vi "FindRouteExample.vi"() -> ()   [LabVIEW 2010]
uses:
  PathTree/RouteTree.lvclass
  Waypoint/point.ctl
  Waypoint/Waypoint.lvclass
panel:
  out "BestTime":u32 caption="Time (ms)"
  out "Best Distance":dbl caption="Distance"
  in  "Best Solve":bool
  out "SmartTime":u32 caption="Time (ms)"
  out "Smart Distance":dbl caption="Distance"
  in  "Smart Solve":bool
  out "FastTime":u32 caption="Time (ms)"
  out "Fast Distance":dbl caption="Distance"
  in  "Fast Solve":bool
  in  "NumPoints":i32
  in  "NewPoints":bool
  in  "Exit":bool
  out "Paths":picture
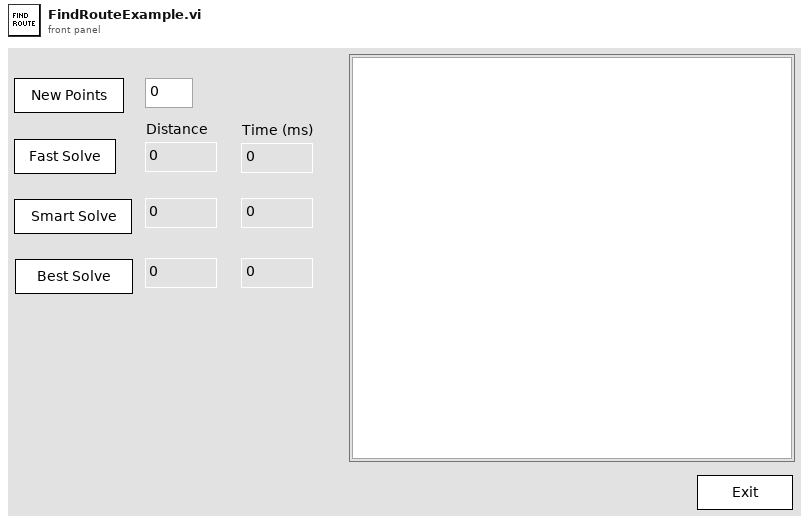
[diagram p1: front panel]
types:
  T1 = typedef "Waypoint.lvclass/point.ctl" = cluster{"X":dbl, "Y":dbl}
  T2 = cluster{"Width":u16, "Style":enum32{"Solid", "Dash", "Dot", "DashDot", "DashDotDot"}}
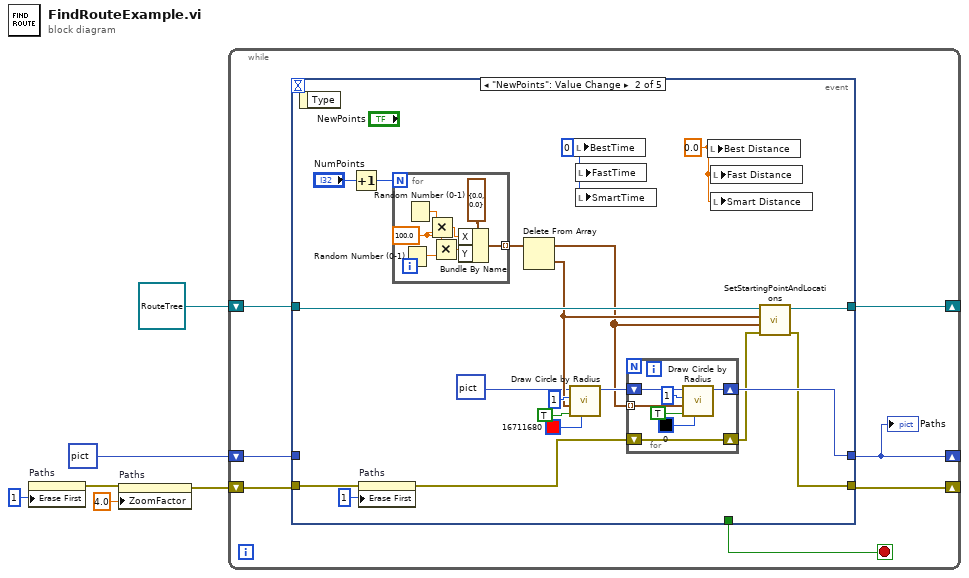
[diagram p0: block diagram]
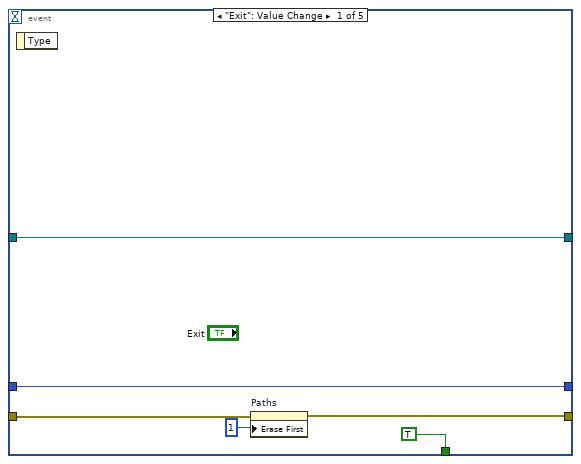
[diagram p2: hidden frame]
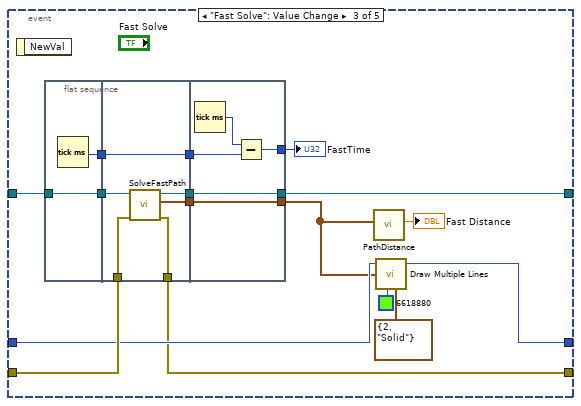
[diagram p3: hidden frame]
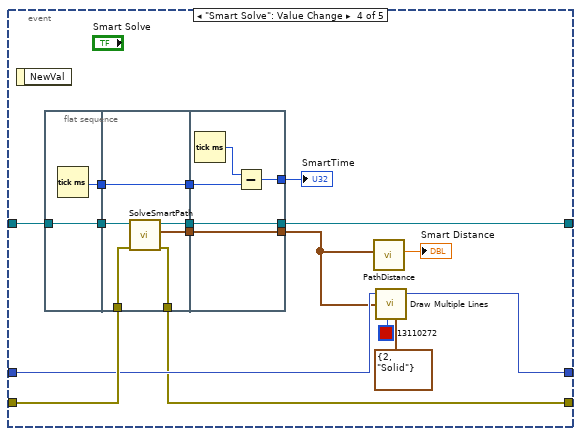
[diagram p4: hidden frame]
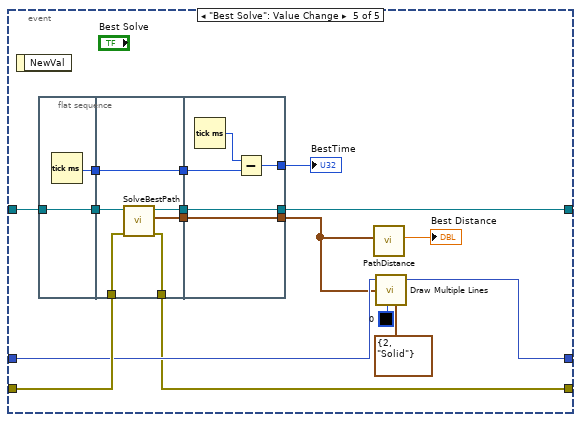
[diagram p5: hidden frame]
diagram:
  n1 = property on="Paths" class="Pict"("Erase First"=u8 1) -> (error out=w1:errorcluster)  [unwired: 2 in, 1 out]
  n2 = property on="Paths" class="Pict"(error in=w1, "ZoomFactor"=sgl 4.0 ("Zoom Factor")) -> (error out=w4:errorcluster)  [unwired: 1 in, 1 out]
  n3 = while {
    shift-right: [w7] -> _
    shift-left: picture data[5B] ("Paths") -> [w10]
    shift-right: [w8] -> _
    shift-left: w4 -> [w9]
    shift-right: [w12] -> _
    shift-left: refnum<class "RouteTree.lvclass"> refnum ("RouteTree.lvclass") -> [w13]
    stop <- w11 stop-if-true
    n4 = event shown="[1] \"NewPoints\": Value Change" {
      selector: _ -> [_ _ _ _ _]
      dyn-events: _ -> [_ _ _ _ _]
      timeout: _ -> [_ _ _ _ _]
      tunnel: w13 -> [w19 w28 w69 w98 w127]
      tunnel: [w19 w27 w68 w97 w126] -> w12
      tunnel: [TRUE _ _ _ _] -> w11
      tunnel: w10 -> [w17 _ w66 w95 w124]
      tunnel: [w17 w29 w63 w92 w121] -> w7
      tunnel: w9 -> [w16 w31 w67 w96 w125]
      tunnel: [w14 w23 w62 w91 w120] -> w8
      event "Exit": Value Change {
        n5 = event-data() -> ()  [unwired: 1 in, 1 out]
        n6 = property on="Paths" class="Pict"(error in=w16, "Erase First"=u8 1) -> (error out=w14:errorcluster)  [unwired: 1 in, 1 out]
      }
      event "NewPoints": Value Change {
        w20 = 0.0 ("Best Distance")
        w21 = u32 0 ("BestTime")
        n7 = event-data() -> ()  [unwired: 1 in, 1 out]
        n8 = Increment(x="NumPoints") -> (x+1=w39:i32)
        n9 = property on="Paths" class="Pict"(error in=w31, "Erase First"=u8 1) -> (error out=w30:errorcluster)  [unwired: 1 in, 1 out]
        n10 = for {
          N: w39 -> [_]
          tunnel: [w47] -> w37 mode=indexing
          w49 = 100.0 ("x")
          n11 = Random Number (0-1)() -> (number: 0 to 1=w51:dbl)
          n12 = Random Number (0-1)() -> (number: 0 to 1=w53:dbl)
          n13 = Multiply(x=w53, y=w49) -> (x*y=w52:dbl)
          n14 = Multiply(x=w49, y=w51) -> (x*y=w50:dbl)
          n15 = Bundle By Name(cluster=T1 {"X"=0.0, "Y"=0.0} ("point"), "X"=w52, "Y"=w50) -> (w47:T1)
        }
        n16 = Delete From Array(array=w37) -> (deleted portion=w26:T1, array with subset deleted=w25:T1[])  [unwired: 2 in]
        n17 = call <vilib>:"Draw Circle by Radius.vi"("color(black)"=u32 16711680, "fill?(F)"=TRUE, "pixel center"=w26, "radius"=i16 1, "picture"=picture data[5B]) -> ("new picture"=w33:picture)  [unwired: 6 in]
        n18 = local write "BestTime"(w21) -> ()
        n19 = local write "FastTime"(w21) -> ()
        n20 = local write "SmartTime"(w21) -> ()
        n21 = for {
          shift-right: [w42] -> w29
          shift-left: w33 -> [w43]
          shift-right: [w41] -> w24
          shift-left: w30 -> [w41]
          tunnel: w25 -> [w40] mode=indexing
          n22 = call <vilib>:"Draw Circle by Radius.vi"("color(black)"=u32 0, "fill?(F)"=TRUE, "pixel center"=w40, "radius"=i16 1, "picture"=w43) -> ("new picture"=w42:picture)  [unwired: 6 in]
        }
        n23 = local write "Best Distance"(w20) -> ()
        n24 = local write "Fast Distance"(w20) -> ()
        n25 = local write "Smart Distance"(w20) -> ()
        n26 = call "SetStartingPointAndLocations.vi"("error in (no error)"=w24, "locations"=w25, "point"=w26, "PathTree in"=w28) -> ("error out"=w23:errorcluster, "PathTree out"=w27:refnum<class "RouteTree.lvclass">)  [unwired: 6 in]
      }
      event "Fast Solve": Value Change {
        n27 = event-data() -> ()  [unwired: 1 in, 1 out]
        n28 = flat-sequence {
          tunnel: w69 -> [w71]
          tunnel: [w71] -> w57
          tunnel: [w70] -> w56
          tunnel: w67 -> [w75]
          tunnel: [w74] -> w62
          tunnel: [w76] -> w59
          tunnel: [w73] -> w58
          tunnel: w57 -> [w77]
          tunnel: w56 -> [w72]
          tunnel: [w72] -> w55
          tunnel: [w81] -> w61
          tunnel: [w82] -> w68
          tunnel: w59 -> [w82]
          tunnel: w58 -> [w81]
          tunnel: w55 -> [w79]
          tunnel: [w78] -> w54
          frame #0 {
            n29 = Tick Count (ms)() -> (millisecond timer value=w70:u32)
          }
          frame #1 {
            n30 = call "SolveFastPath.vi"("error in (no error)"=w75, "RouteTree in"=w77) -> ("error out"=w74:errorcluster, "greedy Path"=w73:T1[], "RouteTree out"=w76:refnum<class "RouteTree.lvclass">)  [unwired: 7 in]
          }
          frame #2 {
            n31 = Tick Count (ms)() -> (millisecond timer value=w80:u32)
            n32 = Subtract(x=w80, y=w79) -> (x-y=w78:u32)
          }
        }
        n33 = call "PathDistance.vi"("path"=w61) -> ("distance"=→"Fast Distance":dbl)  [unwired: 10 in]
        n34 = call <vilib>:"Draw Multiple Lines.vi"("picture"=w66, "line endpoints"=w61, "color(black)"=u32 6618880, "pen"=T2 {"Width"=2, "Style"=enum."Solid"}) -> ("new picture"=w63:picture)  [unwired: 5 in]
        "FastTime" <- w54
      }
      event "Smart Solve": Value Change {
        n35 = event-data() -> ()  [unwired: 1 in, 1 out]
        n36 = flat-sequence {
          tunnel: w98 -> [w100]
          tunnel: [w100] -> w87
          tunnel: [w99] -> w86
          tunnel: w96 -> [w104]
          tunnel: [w103] -> w91
          tunnel: [w105] -> w89
          tunnel: [w102] -> w88
          tunnel: w87 -> [w106]
          tunnel: w86 -> [w101]
          tunnel: [w101] -> w85
          tunnel: [w110] -> w90
          tunnel: [w111] -> w97
          tunnel: w89 -> [w111]
          tunnel: w88 -> [w110]
          tunnel: w85 -> [w108]
          tunnel: [w107] -> w84
          frame #0 {
            n37 = Tick Count (ms)() -> (millisecond timer value=w99:u32)
          }
          frame #1 {
            n38 = call "SolveSmartPath.vi"("error in (no error)"=w104, "RouteTree in"=w106) -> ("error out"=w103:errorcluster, "Best First Path"=w102:T1[], "RouteTree out"=w105:refnum<class "RouteTree.lvclass">)  [unwired: 6 in, 1 out]
          }
          frame #2 {
            n39 = Tick Count (ms)() -> (millisecond timer value=w109:u32)
            n40 = Subtract(x=w109, y=w108) -> (x-y=w107:u32)
          }
        }
        n41 = call "PathDistance.vi"("path"=w90) -> ("distance"=→"Smart Distance":dbl)  [unwired: 10 in]
        n42 = call <vilib>:"Draw Multiple Lines.vi"("picture"=w95, "line endpoints"=w90, "color(black)"=u32 13110272, "pen"=T2 {"Width"=2, "Style"=enum."Solid"}) -> ("new picture"=w92:picture)  [unwired: 5 in]
        "SmartTime" <- w84
      }
      event "Best Solve": Value Change {
        n43 = event-data() -> ()  [unwired: 1 in, 1 out]
        n44 = flat-sequence {
          tunnel: w127 -> [w129]
          tunnel: [w129] -> w116
          tunnel: [w128] -> w115
          tunnel: w125 -> [w133]
          tunnel: [w132] -> w120
          tunnel: [w134] -> w118
          tunnel: [w131] -> w117
          tunnel: w116 -> [w135]
          tunnel: w115 -> [w130]
          tunnel: [w130] -> w114
          tunnel: [w140] -> w119
          tunnel: [w136] -> w126
          tunnel: w118 -> [w136]
          tunnel: w117 -> [w140]
          tunnel: w114 -> [w138]
          tunnel: [w137] -> w113
          frame #0 {
            n45 = Tick Count (ms)() -> (millisecond timer value=w128:u32)
          }
          frame #1 {
            n46 = call "SolveBestPath.vi"("error in (no error)"=w133, "RouteTree in"=w135) -> ("error out"=w132:errorcluster, "Path"=w131:T1[], "RouteTree out"=w134:refnum<class "RouteTree.lvclass">)  [unwired: 6 in, 1 out]
          }
          frame #2 {
            n47 = Tick Count (ms)() -> (millisecond timer value=w139:u32)
            n48 = Subtract(x=w139, y=w138) -> (x-y=w137:u32)
          }
        }
        n49 = call "PathDistance.vi"("path"=w119) -> ("distance"=→"Best Distance":dbl)  [unwired: 10 in]
        n50 = call <vilib>:"Draw Multiple Lines.vi"("picture"=w124, "line endpoints"=w119, "color(black)"=u32 0, "pen"=T2 {"Width"=2, "Style"=enum."Solid"}) -> ("new picture"=w121:picture)  [unwired: 5 in]
        "BestTime" <- w113
      }
    }
    "Paths" <- w7
  }
